vi "Command Turn to Heading Tighter.vi"(7 "Startup":bool, 9 "Timeout":dbl=15.0, 11 "Heading":dbl=-90.0) -> (2 "Right Wheel Velocity":dbl=680.96, 3 "Left Wheel Velocity":dbl=-680.96, 4 "Reint":bool, 6 "Completed":bool)   [LabVIEW 2017]
uses:
  Command Execution State.ctl
  Utility VIs/Refnum Names.vi
  <vilib>/Rock Robotics/WPI/ThirdParty/Phoenix-LabVIEW/Pigeon IMU/CTRE_PigeonIMU_GetRawGyro.vi
  Drive/Drive Globals.vi
panel:
  out "Using Lower?":bool=TRUE
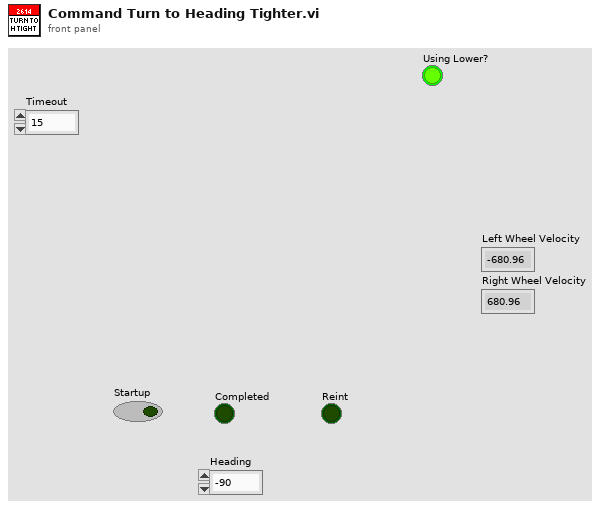
[diagram p1: front panel]
types:
  T1 = typedef "Command Execution State.ctl" = enum16{"Initialize", "Execute", "Finish"}
  T2 = typedef "CTRE_PigeonIMU_DeviceRef.ctl" = cluster{"DeviceStatus":errorcluster, "Device Number":u8, "Type":T3, "Device ID":u32, "Handle":u64, "UsageFrame":u32, "Library Path":path}
  T3 = typedef "CTRE_PigeonIMU_ConnectionType.ctl" = u32
  T4 = cluster{"X":dbl, "Y":dbl, "Z":dbl, "Magnitude":dbl}
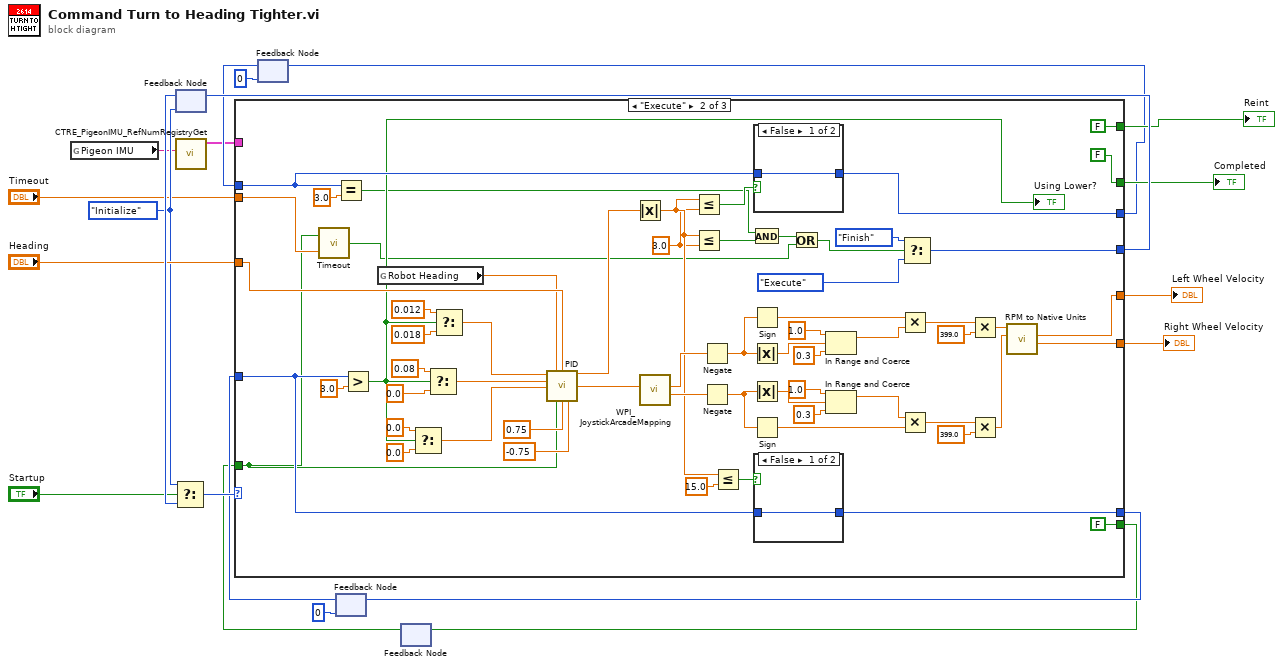
[diagram p0: block diagram]
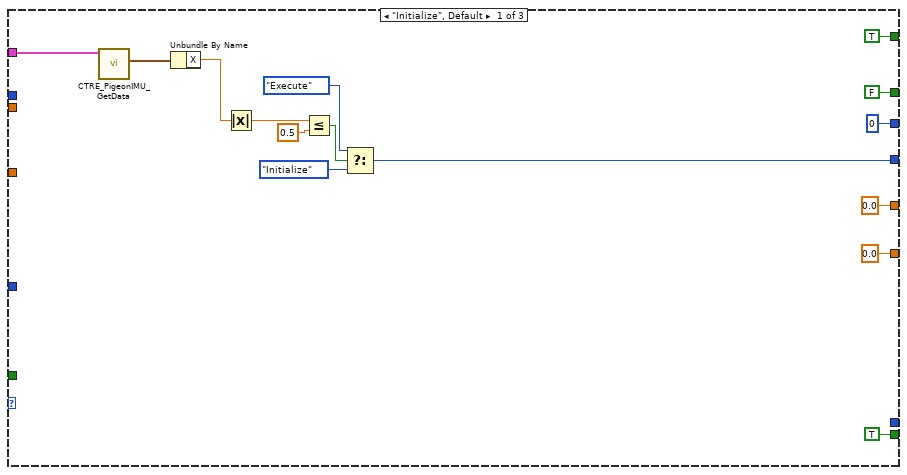
[diagram p2: hidden frame]
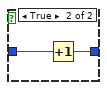
[diagram p3: hidden frame]
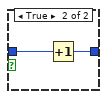
[diagram p4: hidden frame]
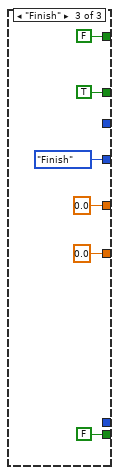
[diagram p5: hidden frame]
diagram:
  w17 = Command_Execution_State."Initialize" ("Play State")
  n1 = global read "Refnum Names.vi" "Pigeon IMU"() -> (w8:string)
  n2 = feedback #1(w17) -> (w19:T1)
  n3 = Select(t=w17, s="Startup", f=w19) -> (s? t:f=w21:T1)
  n4 = call <vilib>:"CTRE_PigeonIMU_RefNumRegistryGet.vi"("refnum name"=w8) -> ("PigeonIMUDevRef"=w7:T2)  [unwired: 9 in, 1 out]
  n5 = feedback #2(0) -> (w10:i32)
  n6 = feedback #3(0 ("y")) -> (w6:i32)
  n7 = feedback #4() -> (w1:bool)  [unwired: 1 in]
  n8 = case shown="\"Execute\"" w21 {
    tunnel: [w28 w95 Command_Execution_State."Finish" ("Play State")] -> w20
    tunnel: "Heading" -> [_ w92 _]
    tunnel: [FALSE FALSE TRUE] -> w16
    tunnel: [TRUE FALSE FALSE] -> w14
    tunnel: [0.0 w49 0.0] -> w13
    tunnel: [0.0 w48 0.0] -> w12
    tunnel: w10 -> [_ w83 _]
    tunnel: [0 w84 _] -> w9
    tunnel: w7 -> [w30 _ _]
    tunnel: w6 -> [_ w70 _]
    tunnel: [_ w71 _] -> w5
    tunnel: "Timeout" -> [_ w55 _]
    tunnel: [TRUE FALSE FALSE] -> w2
    tunnel: w1 -> [_ w37 _]
    frame "Initialize", Default {
      n9 = call-poly <vilib>:"CTRE_PigeonIMU_GetData.vi"("PigeonIMUDevRef"=w30) -> ("Gyro DPS"=w31:T4)  [unwired: 8 in, 2 out]
      n10 = Unbundle By Name(w31) -> ("X"=w27:dbl)
      n11 = Absolute Value(x=w27) -> (abs(x)=w25:dbl)
      n12 = Less Or Equal?(x=w25, y=0.5) -> (x <= y?=w24:bool)
      n13 = Select(t=Command_Execution_State."Execute" ("Play State"), s=w24, f=Command_Execution_State."Initialize") -> (s? t:f=w28:T1)
    }
    frame "Execute" {
      w46 = 3.0 ("t")
      n14 = call "Timeout.vi"("Timeout"=w55, "Initialize"=w37) -> ("Timed Out?"=w53:bool)
      n15 = Equal?(x=w83, y=3.0 ("t")) -> (x = y?=w76:bool)
      n16 = Greater?(x=w70, y=3.0 ("t")) -> (0:w77:bool)
      "Using Lower?" <- w77
      n17 = global read "Drive Globals.vi" "Robot Heading"() -> (w91:dbl)
      n18 = Select(t=0.0, s=w77, f=0.0 ("t")) -> (s? t:f=w79:dbl)
      n19 = Select(t=0.08, s=w77, f=0.0 ("t")) -> (s? t:f=w78:dbl)
      n20 = Select(t=0.012, s=w77, f=0.018 ("t")) -> (s? t:f=w80:dbl)
      n21 = call "PID.vi"("Kp"=w80, "Process Variable"=w91, "Goal"=w92, "Ki"=w78, "Kd"=w79, "Reinit"=w37, "Max Ouput"=0.75, "Min Output"=-0.75) -> ("Current Error"=w93:dbl, "Command"=w89:dbl)  [unwired: 5 in, 1 out]
      n22 = Absolute Value(x=w93) -> (abs(x)=w73:dbl)
      n23 = call <vilib>:"WPI_JoystickArcadeMapping.vi"("X axis value"=w89) -> ("Right Motor Value"=w87:dbl, "Left Motor Value"=w88:dbl)  [unwired: 9 in]
      n24 = Less Or Equal?(x=w73, y=w46) -> (x <= y?=w90:bool)
      n25 = Less Or Equal?(x=w73, y=w46) -> (x <= y?=w74:bool)
      n26 = Negate(x=w88) -> (-x=w59:dbl)
      n27 = Negate(x=w87) -> (-x=w58:dbl)
      n28 = Less Or Equal?(x=w73, y=15.0 ("t")) -> (x <= y?=w72:bool)
      n29 = And(x=w76, y=w74) -> (x .and. y?=w75:bool)
      n30 = Sign(1:w59) -> (0:w67:dbl)
      n31 = Absolute Value(x=w59) -> (abs(x)=w69:dbl)
      n32 = Absolute Value(x=w58) -> (abs(x)=w68:dbl)
      n33 = Sign(1:w58) -> (0:w64:dbl)
      n34 = case shown="False" w90 {
        tunnel: w83 -> [w102 w104]
        tunnel: [w102 w103] -> w84
        frame False {
        }
        frame True {
          n35 = Increment(x=w104) -> (x+1=w103:i32)
        }
      }
      n36 = case shown="False" w72 {
        tunnel: w70 -> [w99 w101]
        tunnel: [w99 w100] -> w71
        frame False {
        }
        frame True {
          n37 = Increment(x=w101) -> (x+1=w100:i32)
        }
      }
      n38 = Or(x=w75, y=w53) -> (x .or. y?=w54:bool)
      n39 = In Range and Coerce(upper limit=1.0, x=w69, lower limit=0.3) -> (coerced(x)=w66:dbl)  [unwired: 1 out]
      n40 = In Range and Coerce(upper limit=1.0, x=w68, lower limit=0.3) -> (coerced(x)=w65:dbl)  [unwired: 1 out]
      n41 = Multiply(x=w67, y=w66) -> (x*y=w56:dbl)
      n42 = Multiply(x=w65, y=w64) -> (x*y=w57:dbl)
      n43 = Select(t=Command_Execution_State."Finish" ("Play State"), s=w54, f=Command_Execution_State."Execute") -> (s? t:f=w95:T1)
      n44 = Multiply(x=w56, y=399.0) -> (x*y=w51:dbl)
      n45 = Multiply(x=w57, y=399.0) -> (x*y=w50:dbl)
      n46 = call "RPM to Native Units.vi"("Right RPM"=w50, "Left RPM"=w51) -> ("Right Out"=w48:dbl, "Left Out"=w49:dbl)  [unwired: 6 in, 1 out]
    }
    frame "Finish" {
    }
  }
  "Completed" <- w16
  "Reint" <- w14
  "Left Wheel Velocity" <- w13
  "Right Wheel Velocity" <- w12
  n47 = feedback-in #1(w20) -> ()
  n48 = feedback-in #2(w9) -> ()
  n49 = feedback-in #3(w5) -> ()
  n50 = feedback-in #4(w2) -> ()
